vi "Cal Inst - Settings.vi"(8 "error in (no error)":errorcluster, 11 "Data Cluster":T1={"VISA Refnum in"="", "Serial Configuration"={"Baud Rate"=0, "Flow Control"=0}, "Voltage Level (0V)"=0.0, "Output Phase(s) (1-Phase)"=0, "Active Phase (1:Phase 1)"=1} {"Output Phase(s) (1-Phase)" items=["3 phase", "1 phase"]; "Active Phase (1:Phase 1)" items=["Phase 1"=1, "Phase 2"=2, "Phase 3"=3]; "Serial Configuration"."Flow Control" items=["None", "XON/XOFF", "RTS/CTS", "XON/XOFF & RTS/CTS", "DTR/DSR", "XON/XOFF & DTR/DSR"]; "Serial Configuration"."Baud Rate" items=["9600"=9600, "19200"=19200, "38400"=38400, "57600"=57600, "115200"=115200, "230400"=230400, "460800"=460800]}) -> (0 "error out":errorcluster)   [LabVIEW 2013, in "Cal Inst.lvlib"]
uses:
  Hardware Configuration.ctl
  Cal Inst.lvlib
  Libraries/California Instruments iX Series/California Instruments iX Series.lvlib
  Cal Inst Acquisition.lvlib
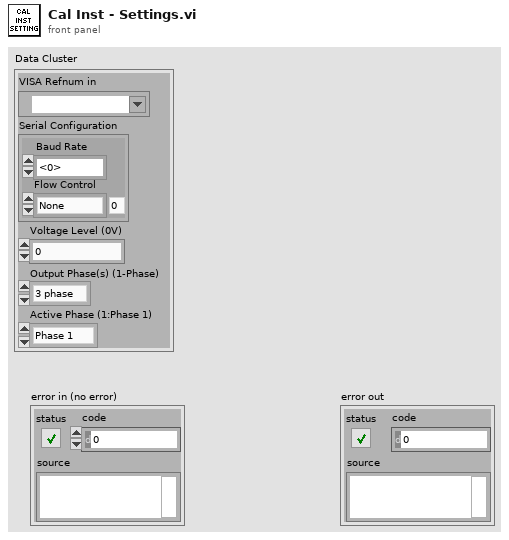
[diagram p1: front panel]
types:
  T1 = typedef "Cal Inst.lvlib/Cal Inst Acquisition.lvlib/Hardware Configuration.ctl" = cluster{"VISA Refnum in":refnum<visa-resource-name>, "Serial Configuration":cluster{"Baud Rate":u32, "Flow Control":u16}, "Voltage Level (0V)":dbl, "Output Phase(s) (1-Phase)":u16, "Active Phase (1:Phase 1)":i32}
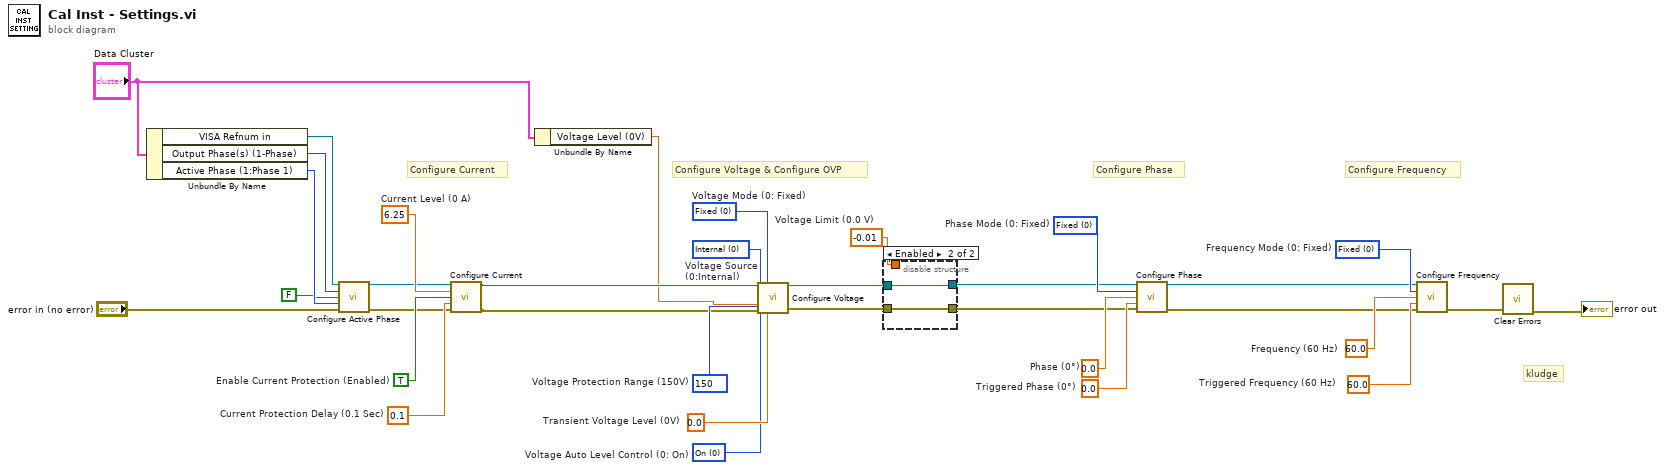
[diagram p0: block diagram]
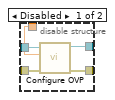
[diagram p2: hidden frame]
diagram:
  w20 = 60.0  # Triggered Frequency (60 Hz)
  w19 = 60.0  # Frequency (60 Hz)
  w18 = 0 items=["Fixed", "Step", "Pulse", "List", "Sense", "External"]  # Frequency Mode (0: Fixed)
  w23 = 0.0  # Triggered Phase (0°)
  w22 = 0.0  # Phase (0°)
  w21 = 0 items=["Fixed", "Step", "Pulse", "List"]  # Phase Mode (0: Fixed)
  w31 = -0.01  # Voltage Limit (0.0 V)
  w28 = u16 150 items=["150"=150, "300"=300]  # Voltage Protection Range (150V)
  w25 = u16 0 items=["On", "Off", "Regulation"]  # Voltage Auto Level Control (0: On)
  w26 = u16 0 items=["Internal", "External"]  # Voltage Source (0:Internal)
  w24 = 0 items=["Fixed", "Step", "Pulse", "List"]  # Voltage Mode (0: Fixed)
  w27 = 0.0  # Transient Voltage Level (0V)
  w34 = 0.1  # Current Protection Delay (0.1 Sec)
  w33 = TRUE  # Enable Current Protection (Enabled)
  w32 = 6.25  # Current Level (0 A)
  # "kludge"
  # "Configure Frequency"
  # "Configure Phase"
  # "Configure Voltage & Configure OVP"
  # "Configure Current"
  n1 = Unbundle By Name("Data Cluster") -> ("VISA Refnum in"=w6:refnum<visa-resource-name>, "Output Phase(s) (1-Phase)"=w5:u16, "Active Phase (1:Phase 1)"=w4:i32)
  n2 = call "Configure Active Phase.vi"("VISA resource name"=w6, "Output Phase(s) (3-Phase)"=w5, "Enable Coupling (Enabled)"=FALSE, "Active Phase (1:Phase 1)"=w4, "error in (no error)"="error in (no error)") -> ("VISA resource name out"=w7:refnum<visa-resource-name>, "error out"=w8:errorcluster)  [unwired: 9 in]
  n3 = call "Configure Current.vi"("VISA resource name"=w7, "Current Level (0 A)"=w32, "Enable Current Protection (Enabled)"=w33, "Current Protection Delay (0.1 Sec)"=w34, "error in (no error)"=w8) -> ("VISA resource name out"=w17:refnum<visa-resource-name>, "error out"=w16:errorcluster)  [unwired: 9 in]
  n4 = Unbundle By Name("Data Cluster") -> ("Voltage Level (0V)"=w11:dbl)
  n5 = call "Configure Voltage.vi"("VISA resource name"=w17, "Voltage Mode (0: Fixed)"=w24, "Voltage Auto Level Control (0: On)"=w25, "Voltage Source (0:Internal)"=w26, "Voltage Level (0V)"=w11, "error in (no error)"=w16, "Transient Voltage Level (0V)"=w27, "Voltage Protection Range (150V)"=w28) -> ("VISA resource name out"=w29:refnum<visa-resource-name>, "error out"=w30:errorcluster)  [unwired: 6 in]
  n6 = disable-structure shown="Enabled" {
    disable-tunnel: w29 -> [w39 w41]
    disable-tunnel: w30 -> [w38 w40]
    disable-tunnel: w31 -> [w37 _]
    disable-tunnel: [w36 w41] -> w15
    disable-tunnel: [w35 w40] -> w14
    frame Disabled {
      n7 = call "Configure OVP.vi"("error in (no error)"=w38, "Voltage Limit (0.0 V)"=w37, "VISA resource name"=w39) -> ("error out"=w35:errorcluster, "VISA resource name out"=w36:refnum<visa-resource-name>)  [unwired: 7 in]
    }
    frame Enabled {
    }
  }
  n8 = call "Configure Phase.vi"("VISA resource name"=w15, "Phase Mode (0: Fixed)"=w21, "Phase (0°)"=w22, "Triggered Phase (0°)"=w23, "error in (no error)"=w14) -> ("VISA resource name out"=w13:refnum<visa-resource-name>, "error out"=w12:errorcluster)  [unwired: 9 in]
  n9 = call "Configure Frequency.vi"("VISA resource name"=w13, "Frequency Mode (0: Fixed)"=w18, "Frequency (60 Hz)"=w19, "Triggered Frequency (60 Hz)"=w20, "error in (no error)"=w12) -> ("error out"=w3:errorcluster)  [unwired: 9 in, 1 out]
  n10 = call <vilib>:"Clear Errors.vi"("error in (no error)"=w3) -> ("error out"=→"error out":errorcluster)  [unwired: 6 in]
